vi "SendBroadcastMessage.vi"(8 "error in (no error)":errorcluster, 9 "message value":variant, 10 "message name":string, 11 "Qbus in":refnum<class "Qbus.lvclass">) -> (0 "error in (no error)":errorcluster, 3 "Qbus out":refnum<class "Qbus.lvclass">)   [LabVIEW 2017, in "Qbus.lvclass"]
doc: "Sends a Qbus message to any process that is subscribed to that type of message."
uses:
  <vilib>/addons/Qbus/Qbus.lvclass
  <vilib>/addons/Qbus/Qbus.lvclass/Qbus.ctl
  <vilib>/addons/Qbus/controls/message.ctl
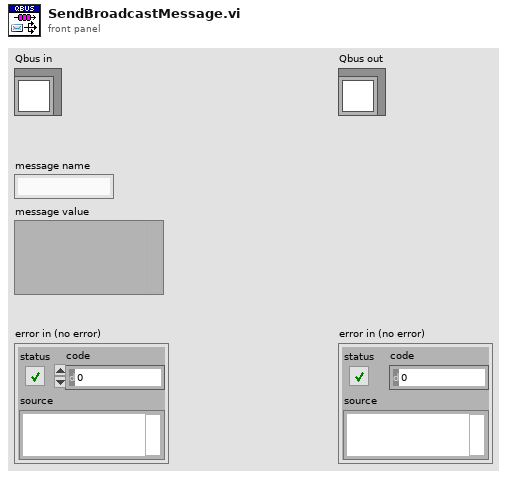
[diagram p1: front panel]
types:
  T1 = typedef "Qbus.lvclass/message.ctl" = cluster{"MsgName":string, "MsgValue":variant}
  T2 = typedef "Qbus.lvclass/data.ctl" = cluster{"Queues":variant, "Subscriptions":variant, "MasterQ":string}
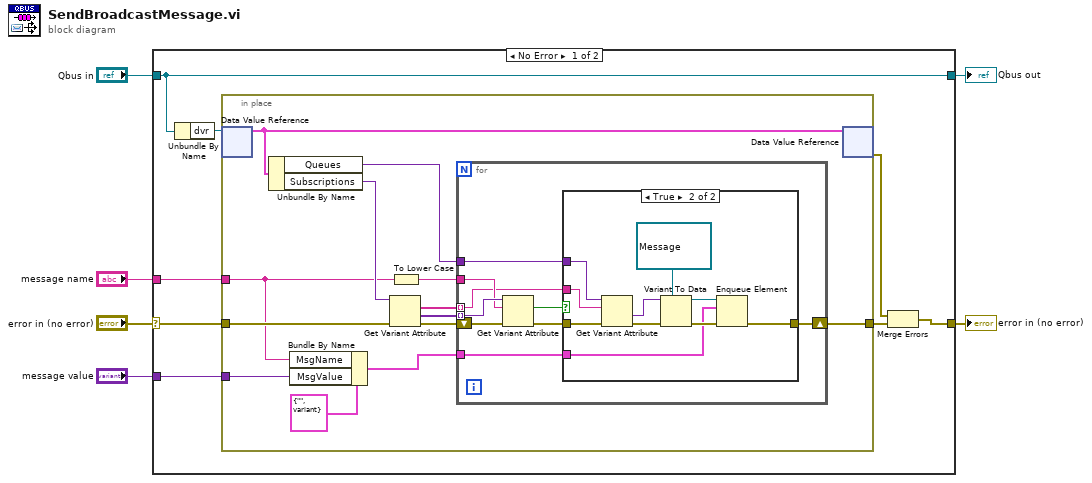
[diagram p0: block diagram]
diagram:
  n1 = case shown="No Error" "error in (no error)" {
    selector: "error in (no error)" -> [w11 w49]
    tunnel: [w10 w49] -> w5
    tunnel: [w14 w48] -> w3
    tunnel: "Qbus in" -> [w14 w48]
    tunnel: "message name" -> [w8 _]
    tunnel: "message value" -> [w7 _]
    frame No Error {
      n2 = Unbundle By Name(w14) -> ("dvr"=w13:refnum<data-value>)
      n3 = in-place {
        in-place-border: w11 -> [w27]
        in-place-border: [w20] -> w9
        in-place-border: w8 -> [w17]
        in-place-border: w7 -> [w16]
        n4 = in-place-dvr #1(w13) -> (w25:T2)  [unwired: 1 out]
        n5 = Unbundle By Name(w25) -> ("Queues"=w19:variant, "Subscriptions"=w26:variant)
        n6 = Bundle By Name(cluster=T1 {"MsgName"="", "MsgValue"=variant} ("Message"), "MsgName"=w17, "MsgValue"=w16) -> (w15:T1)
        n7 = Get Variant Attribute(Variant=w26, error in=w27) -> (names=w24:string[], values=w22:variant[], error out=w21:errorcluster)  [unwired: 2 in, 1 out]
        n8 = To Lower Case(string=w17) -> (all lower case string=w23:string)
        n9 = for {
          tunnel: w24 -> [w29] mode=indexing
          tunnel: w23 -> [w33]
          tunnel: w22 -> [w35] mode=indexing
          shift-right: [w36] -> w20
          shift-left: w21 -> [w34]
          tunnel: w19 -> [w30]
          tunnel: w15 -> [w28]
          n10 = Get Variant Attribute(Variant=w35, name=w33, error in=w34) -> (found=w32:bool, error out=w31:errorcluster)  [unwired: 1 in, 2 out]
          n11 = case shown="True" w32 {
            tunnel: w31 -> [w37 w44]
            tunnel: [w37 w45] -> w36
            tunnel: w30 -> [_ w43]
            tunnel: w29 -> [_ w42]
            tunnel: w28 -> [_ w38]
            frame False {
            }
            frame True {
              n12 = Get Variant Attribute(Variant=w43, name=w42, error in=w44) -> (value=w41:variant, error out=w40:errorcluster)  [unwired: 1 in, 2 out]
              n13 = Variant To Data(error in=w40, type=refnum<queue> refnum ("queue out"), Variant=w41) -> (data=w39:refnum<queue>, error out=w46:errorcluster)
              n14 = Enqueue Element(queue=w39, element=w38, error in (no error)=w46) -> (error out=w45:errorcluster)  [unwired: 1 in, 2 out]
            }
          }
        }
        n15 = in-place-dvr #1(w25) -> (w12:errorcluster)  [unwired: 1 out]
      }
      n16 = Merge Errors(w12, w9) -> (w10:errorcluster)
    }
    frame Error {
    }
  }
  "error in (no error)" <- w5
  "Qbus out" <- w3
